vi "HFRR ADV v07.vi"() -> ()   [LabVIEW 2025] (continued)
]]
  out "Residual Uno":string
  out "Residual Due":string
  out "String":string="C:\\Winducom 2010\\1582\\1582\\"
  out "file path":path=path "C:/Windows/wndcm_pw_stdED hfrr.txt"
  out "string":string="49\r50\r51\r10"
  out "x = y?":bool
  out "dipl pwd":string="@143$\n"
  out "string1 4":string
  out "string1 3":string
  out "string1 2":string
  out "string1":string
  out "stopT":bool
  out "Elapsed time 3":dbl=0.10620016403198242 min=0.0 max=6000.0 step=0.01 format="%<%H:%M:%S>t"
  in  "error in (no error)":errorcluster
  out "error out":errorcluster
  in  "RSTCOF 2":bool
  out "PID output":dbl=42.16277107130474 format="%.2f"
  out "Flag":dbl format="%.2f"
  in  "Tab Control 3":enum32{"RMS", "LIVE"}(tab)
  out "array w/ subset deleted":dbl[](array[numeric])
  out "REMARKS":string="@WINDUCOM : RECIPROCATORY TEST RIG    DEFINITON FILE       \r  Sample ID :- , Load :-  2.00 N , Remarks :- , Date :- 05/11/2016, 06:04\r"
  out "Time 2":dbl=0.0004
  in  "reinit":bool=TRUE
  in  "Remarks : 2":string
  out "PID-out":dbl
  out "Rate":dbl=2500.0 caption="Rate (Hz)" min=100.0 max=10000.0 step=1.0
  out "COUNT":i32
  out "FRICVALZ":dbl
  out "Sensor mean 3":dbl
  out "Sensor mean":dbl(slide) min=0.0 max=5.0 step=0.001 scale=0.0..5.0
  out "Sensor mean 2":dbl
  in  "ao0":errorcluster
  out "String 2":string
  out "clk":dbl min=0.0 max=999999999.0 step=0.25 format="%.2f"
  out "spm":string
  out "stp":dbl=0.25 min=0.25 max=60.0 step=0.25 format="%.2f"
  # "© Copyright 2023 | Paltro Inc"
  # "HFRR ADV"
  # "ADV"
  # "Camera Initialization in Progress"
  # "Test Setup"
  # "SAMPLE INFO"
  # "Hz"
  # "grams"
  # "mm"
  # "°C"
  # "%RH"
  # "min"
  # "mins remaining"
  # "°C"
  # "Coefficient of Friction"
  # "Frictional Force ( N )"
  # "Electrical Contact Resistance ( % )"
  # "Temperature ( °C )"
  # "Heater"
  # "( mm )"
  # "Hz"
  # "%Rh"
  # "Stroke ( mm )"
  # "Controller"
  # "%"
  # "N"
  # "deg C"
  # "N"
  # "Automated Scar Detection in Progress"
  # "Zoom Factor"
  # "%"
  # "Tools"
  # "Wear Scar Measurements"
  # "Wear Scar"
  # "Wear Scar"
  # "Wear Scar"
  # "µm"
  # "µm"
  # "µm"
  # "Calibration Centre"
  # "Select a calibration procedure to begin. Each procedure guides you through all required steps."
  # "System Control Commands\nS;1 - Starts the full automation cycle (Runs Priming-humidify till 70RH sequence first, then switches to Maintenance).\nS;0 - Stops the system immediately and enters Standby mode (Safe State: All actuators OFF).\nM;1 - Skips the priming sequence and jumps directly to Maintenance mode (PID control).\nR;1 - Resets the logic state machine and clears all errors, returning to Standby.\nService Mode (Manual Control)\nX;1 - Enters Manual Service Mode. This disables all automatic logic, sensor safety checks, and timers.\nX;0 - Exits Manual Service Mode and returns to Standby (Safe State).\nActuator Commands (Only work after sending X;1)\nP;[0-255] - Sets the Pump PWM. Note that this is Active Low (0 = Max Flow, 255 = Pump OFF).\nF;I;[0-255] - Sets the Intake Fan speed (0 = OFF, 255 = Max Speed).\nF;O;[0-255] - Sets the Exhaust Fan speed (0 = OFF, 255 = Max Speed).\nD;1 - Turns the Dehumidifier Relay ON.\nD;0 - Turns the Dehumidifier Relay OFF."
  # "%RH"
  # "ISO : WS1.4"
  # "Start test and end test log--- done\nDisable heater ON and Humidity ON during the test --- done\ntemprature and ---done\nhumidity reach log\nauto start run true logic and log\nmanual start log once"
  # "Reference Fluid Information"
  # "Note:\nMake sure to place all images in the folder \"C:\\WinDucom\\im\" before clicking on \"Import Image.\""
  # "NOTE:\nPlace all the images in the path \"C:\\WinDucom\\im\" before clicking on Import Image"
  # "Wear Scar Measurements"
  # "Reference Fluid Information"
  # "Graph :"
types:
  T1 = enum32{"Home", "Dashboard", "Imaging", "Report", "Analysis", "About", "Test Setup", "Advance", "Calibration"}
  T2 = enum32{"HOME", "Test Setup", "Acquire", "Adv Scar", "Adv Scar Report", "Compare Files", "Calibration", "About", "Advance", "Mooha"}
  T3 = enum16{"ASTM D6079", "ISO 12156", "CEC F-096-A-06", "Custom"}
  T4 = enum32{"Dashboard 1", "Dashboard 2", "Dashboard 3"}
  T5 = enum32{"COF", "Friction", "ECR", "Temperature", "Humidity", "Stroke"}
  T6 = enum32{"Coefficient Of Friction", "Air Temperature", "Humidity", "Stroke", "Sample Temperature", "Electrical Contact Resistance", "Frequency", "Air Temp vs Rh"}
  T7 = enum32{"Main Tab", "Stroke Calibration", "Friction Force ", "Temperature Calibration"}
  T8 = enum32{"Stroke Calibration", "Friction Calibration", "Temperature Calibration"}
  T9 = enum32{"Gains", "Configuration Parameters", "Temperature Calibration"}
  T10 = enum32{"Stroke Data", "Temperature Calibration", "Friction Force Raw Data"}
  T11 = enum32{"Temp Variables", "Camera", "WO 2465 (1)", "WO 2465 (2)", "WO 2465 (3)"}
  T12 = typedef "Auto Start enum.ctl" = enum16{"Init", "Humidity & Temperature On", "Reach point", "Maintain Stage", "Start Stage", "close", "Exit"}
  T13 = typedef "imagedata.ctl" = cluster{"image type":i32, "image depth":i32, "image":u8[], "mask":u8[], "colors":u32[], "Rectangle":cluster{"left":i16, "top":i16, "right":i16, "bottom":i16}}
  T14 = enum32{"HOME", "Test Setup", "Acquire", "Compare Files", "Print Report", "About", "Advance", "Mooha"}
  T15 = enum8{"Enabled", "Disabled", "Disabled and Grayed Out"}
  T16 = cluster{"Read Heave and Surge":string, "Bytes at Heave Port":dbl, "Heave and Surge COM Port:":refnum<visa-resource-name>, "Com Port 2":refnum<visa-resource-name>, "Residual Due":string, "Heave COM Status 2":bool, "Heave COM Status":bool, "Port 2":bool, "Sway PPR":dbl, "Surge PPR":dbl, "Heave PPR":dbl, "Sway Pitch":dbl, "Surge Pitch":dbl, "Heave Pitch":dbl, "Sway Pulses/mm":dbl, "Surge Pulses/mm":dbl, "Heave Pulses/mm":dbl, "inner loop":dbl, "Read Heave and Surge 2":string, "String 36":string, "Write S":bool, "WriteCC1":string[], "Heave COM Loop":i32, "LastCom":string, "EXIT":bool, "Error Heave":errorcluster}
  T17 = enum32{"HOME", "Test Setup", "Acquire", "Adv Scar", "Adv Scar Report", "Compare Files", "About", "Advance", "Mooha"}
  T18 = enum16{"Always On", "Always Off", "Off While Running"}
  T19 = typedef "POST ANALYSIS ENUM.ctl" = enum16{"OPEN EXE", "INIT", "OPEN FILE", "FIT", "DRAW REC", "DRAW LINE", "PAN", "ZOOM IN", "ZOOM OUT", "SET ZOOM", "CLEAR ROI", "GET MEASUREMENTS", "RESIZE MODE", "STREAM START", "STREAM STOP", "SHOW UI", "MINIMIZE UI", "HIDE UI", "CKISE APP", "CLOSE CONNECTION", "SAVE IMAGE", "SET ROI COLOR", "READ", "TCP CHECK", "CLOSE"}
  T20 = typedef "CAMERA LIVE FEED ENUM.ctl" = enum16{"OPEN EXE", "INIT", "READ", "CAMERA CONNECT", "CAMERA START", "CAMERA STOP", "CAMERA GRAY", "CAMERA RGB", "CAMERA MINIMIZE", "CAMERA CLOSE", "CAMERA MODE LIST", "CAMERA MODE SET", "CAMERA RESTORE", "CAMERA SAVE", "CLOSE"}
  T21 = cluster{"File Name":string, "Test Method":string, "Operator":string, "Fuel Description":string, "Date and time":string}
  T22 = enum32{"Home", "Dashboard", "Imaging", "Report", "Analysis", "About", "Test Setup"}
  T23 = enum32{"HOME", "Test Setup", "Acquire", "Compare Files", "About", "Advance", "Mooha"}
  T24 = enum16{"deny read/write", "deny write-only", "deny none"}
  T25 = typedef "NI_ReportGenerationCore.lvlib/HTML Report Image Alignment.ctl" = enum16{"(default)", "LEFT", "RIGHT", "TOP", "TEXTTOP", "MIDDLE", "ABSMIDDLE", "BASELINE", "BOTTOM", "ABSBOTTOM"}
  T26 = enum32{"Home", "Dashboard", "Imaging", "Report", "Analysis", "About", "Test Setup", "Advance"}
  T27 = enum16{"open", "replace", "create", "open or create", "replace or create", "replace or create with confirmation"}
  T28 = enum16{"INIT", "READ", "MANUAL WRITE", "WRITE", "CLOSE", "ERROR INIT"}
  T29 = enum16{"open", "open or create", "create or replace", "create", "open (read only)"}
  T30 = cluster{"Mode":enum16{"RTU", "ASCII"}, "Slave Address":u8}
diagram:
  w10 = FALSE ("Visible")
  w11 = T15."Enabled" ("Disabled")
  w14 = FALSE ("Visible")
  w13 = FALSE ("Humidity Off Command")
  w31 = "" ("USER ID")
  (unwired) T17."HOME" ("Main Tab")
  # "[CH1]    - FF\n[CH2]   - TEMPERATURE\n[CH3]    - Humidity\n[CH4]    - AIR TEMP\n[CH5]\\- Visa Uno\n[CH6] \\- Visa Due\n[CH7]  \\- file path\n[CH8]   - Displacement Gain\n[CHA]   - Stroke Gain\n[CHB]   - Stroke PID Gain\n[CHC]   -Language Selection\n[CHD]   -Power +\n[CHE]   -Power_\n[CHF]   -Heater\n[CHG]   -Humidity Wet\n[CHH]   -Humidity Dry\n[CHI]   -Integral Time \n[CHIJ   -Air intercept\n[CHI]   -Temp Intercept"
  n1 = flat-sequence {
    tunnel: [w80] -> w23
    tunnel: w23 -> [w94]
    tunnel: [w93] -> w22
    tunnel: ["ao0"] -> w25
    tunnel: w22 -> [_]
    tunnel: w25 -> [w158]
    tunnel: [w158] -> w24
    tunnel: w24 -> [w204]
    tunnel: [w202] -> w35
    tunnel: [w204] -> w34
    tunnel: w35 -> [w254]
    tunnel: w34 -> [w211]
    tunnel: [w254] -> w21
    tunnel: [w217] -> w20
    tunnel: [w205] -> w19
    tunnel: [w260] -> _
    tunnel: [w259] -> _
    tunnel: [w261] -> w57
    tunnel: w21 -> [w261]
    tunnel: w20 -> [w259]
    tunnel: w19 -> [w260]
    frame #0 {
      n2 = disable-structure shown="Disabled" {
        frame Disabled {
          n3 = control-ref of="This VI"() -> (w68:refnum<vi>)
          n4 = property class="VI"(reference=w68) -> (reference out=w59:refnum<vi>, error out=w63:errorcluster, "Panel"=w67:refnum<vi>)  [unwired: 1 in]
          n5 = property class="Pnl"(reference=w67, error in=w63) -> (reference out=w61:refnum<vi>, error out=w64:errorcluster, "Panes[]"=w66:refnum<vi>[])
          n6 = for {
            tunnel: w66 -> [w74] mode=indexing
            tunnel: T18."Always Off" ("Horizontal Scrollbar Visibility") -> [w73]
            tunnel: w64 -> [w70]
            tunnel: [w69] -> w62
            n7 = property class="Pane"(reference=w74, error in=w70, "HorizScrollbarVisibility"=w73) -> (reference out=w71:refnum<vi>, error out=w72:errorcluster)
            n8 = Close Reference(reference=w71, error in (no error)=w72) -> (error out=w69:errorcluster)
          }
          n9 = Close Reference(reference=w61, error in (no error)=w62) -> (error out=w60:errorcluster)
          n10 = Close Reference(reference=w59, error in (no error)=w60) -> (error out=→"error out 8":errorcluster)
        }
        frame Enabled {
        }
      }
    }
    frame #1 {
      n11 = call "CLOSE CONNECTION.vi"("error in (no error)"="error in (no error) 2") -> ("error out"=w78:errorcluster)  [unwired: 10 in]
      n12 = call <vilib>:"Clear Errors.vi"("error in (no error)"=w78) -> ("error out"=w77:errorcluster)  [unwired: 5 in, 1 out]
      n13 = disable-structure shown="Enabled" {
        disable-tunnel: w77 -> [w84 _]
        disable-tunnel: [w83 _] -> w80
        frame Enabled {
          n14 = call <userlib>:"Fit VI window to Largest Dec.vi"("error in (no error)"=w84, "border spacing (2 px)"=1) -> ("error out"=w87:errorcluster, "dup VI Ref"=w91:refnum<vi>)  [unwired: 4 in]
          n15 = invoke on="Invoke Node" class="VI" method="FP.Run-Time Position.Maximized"(reference=w91, error in=w87) -> (error out=w88:errorcluster)  [unwired: 2 in, 3 out]
          n16 = call <vilib>:"Clear Errors.vi"("error in (no error)"=w88) -> ("error out"=w90:errorcluster)  [unwired: 5 in, 1 out]
          n17 = control-ref of="This VI"() -> (w82:refnum<vi>)
          n18 = invoke on="Invoke Node" class="VI" method="Default Vals.Reinit All"(reference=w82, error in=w90) -> (reference out=w86:refnum<vi>, error out=w85:errorcluster)  [unwired: 1 in, 1 out]
          n19 = Close Reference(reference=w86, error in (no error)=w85) -> (error out=w83:errorcluster)
        }
        frame Disabled {
        }
      }
      n20 = local write "sign in temp"(FALSE ("sign in temp")) -> ()
      n21 = property on="Sign In" class="Bool (strict)"("DisabledEnum"=T15."Disabled" ("Disabled")) -> ()  [unwired: 2 in, 2 out]
      n22 = property on="Auto Scar Check" class="Clust (strict)"("Visible"=TRUE) -> ()  [unwired: 2 in, 2 out]
    }
    frame #2 {
      n23 = call "dialog box.vi"("Status"="Before starting the test, verify that the microscope cable is connected.", "error in"=w94) -> ("error out"=w93:errorcluster)  [unwired: 8 in]
    }
    frame #3 {
      (unwired) T17."HOME" ("Main Tab")
      (unwired) TRUE ("Re-Initialise")
      w100 = FALSE ("Upld AR 2")
      # "kkkkk"
      # "C:\\Windows\\wndcm_pw_stdED hfrr.txt"
      # "C:\\LAB-IQ NXT"
      # "C:\\LAB-IQ NXT\\wndcm_pw_stdED hfrr.txt"
      # "password file"
      n24 = Current VI's Path() -> (path=w113:path)
      n25 = Strip Path(path=w113) -> (stripped path=w106:path)  [unwired: 1 out]
      n26 = Path To String(path=w106) -> (string=w108:string)
      n27 = local write "conststatus"(0.0 ("rpm value : 2")) -> ()
      n28 = local write "Upld AR 2"(TRUE ("Upld AR 2")) -> ()
      n29 = local write "FLAG 2"(0.0 ("FLAG 2")) -> ()
      n30 = local write "Com flag"(u32 0 ("Com flag")) -> ()
      n31 = local write "Lan flag"(0.0 ("Lan flag")) -> ()
      n32 = local write "COUNT"(0 ("COUNT")) -> ()
      n33 = local write "refresh flag"(FALSE ("refresh flag")) -> ()
      n34 = local write "Json St Flg"(w100) -> ()
      n35 = Search/Split String(string=w108, search string/char (-)=".exe") -> (match + rest of string=w110:string)  [unwired: 1 in, 2 out]
      n36 = Match True/False String(2:".vi" ("false string"), 3:".exe" ("true string"), 4:w110) -> (0:w107:bool)  [unwired: 1 out]
      n37 = local write "Json End Flg"(w100) -> ()
      n38 = case shown="True" w107 {
        tunnel: w106 -> [w129 w131]
        tunnel: [w129 w130] -> w104
        frame False {
        }
        frame True {
          n39 = Strip Path(path=w131) -> (stripped path=w130:path)  [unwired: 1 out]
        }
      }
      n40 = Path To String(path=w104) -> (string=→"Gain path":string)
      n41 = local write "Main Tab Display"(T4."Dashboard 1" ("Main Tab Display")) -> ()
      n42 = local write "main tab sub"(enum32{"Page 1", "Page 2"}."Page 1" ("main tab sub")) -> ()
      n43 = local write "Main Tab"(T2."HOME" ("Main Tab")) -> ()
      n44 = local write "EVENT LOG"("") -> ()
      n45 = List Folder(path=path "C:/LAB-IQ" ("directory path"), pattern="*.txt") -> (filenames=w119:string[])  [unwired: 2 in, 3 out]
      n46 = Search 1D Array(1D array=w119, element="wndcm_pw_stdED hfrr.txt") -> (index of element=w122:i32)  [unwired: 1 in]
      n47 = Equal?(x=w122, y=-1) -> (x = y?=w117:bool)
      n48 = case shown="True" w117 {
        frame False {
        }
        frame True {
          n49 = String To Byte Array(string="123\n") -> (unsigned byte array=w136:u8[])
          n50 = Array Size(array=w136) -> (size(s)=w135:i32)
          n51 = for {
            N: w135 -> [_]
            tunnel: w136 -> [w149]
            tunnel: [w146] -> w138 mode=indexing
            tunnel: w135 -> [w141]
            i -> [w139]
            n52 = Decrement(x=w141) -> (x-1=w142:i32)
            n53 = Equal?(x=w139, y=w142) -> (x = y?=w143:bool)
            n54 = Index Array(array=w149, index=w139) -> (element=w148:u8)
            n55 = Number To Decimal String(number=w148) -> (decimal integer string=w147:string)  [unwired: 1 in]
            n56 = Select(t="", s=w143, f="\r") -> (s? t:f=w140:string)
            n57 = Concatenate Strings(w147, w140) -> (w146:string)
          }
          n58 = local read "file path"() -> (w132:path)
          n59 = Concatenate Strings(w138) -> (w134:string)
          n60 = call <vilib>:"Write Characters To File.vi"("append to file? (new file:F)"=FALSE, "character string"=w134, "file path (dialog if empty)"=w132) -> ()  [unwired: 2 in, 1 out]
        }
      }
      n61 = local write "clk"(0.0 ("clk")) -> ()
      n62 = local write "Flag"(0.0 ("Flag")) -> ()
      "file path" <- path "C:/LAB-IQ/wndcm_pw_stdED hfrr.txt" ("file path")
      "FF buffer" <- dbl[] [] ("FF buffer")
    }
    frame #4 {
      # "C:\\WinDucom\\calibrate WO 2391.dcf"
      n63 = String To Path(string="C:\\LAB-IQ\\calibrate WO 2465.dcf") -> (path=w157:path)
      n64 = Open/Create/Replace File "Open File"(file path (use dialog)=w157) -> (refnum out=w156:refnum<file>)  [unwired: 5 in, 2 out]
      n65 = for {
        N: 24 -> [_]
        tunnel: w156 -> [w177]
        i -> [w171]
        (unwired) TRUE ("line mode (F)")
        n66 = Read from Text File "Read File"(file (use dialog)=w177) -> (text=w176:string)  [unwired: 3 in, 3 out]
        n67 = Match Pattern(string=w176, regular expression="]") -> (after substring=w174:string)  [unwired: 1 in, 3 out]
        n68 = String Subset(string=w176, offset (0)=5, length (rest)=10 ("length (rest)")) -> (substring=w169:string)
        n69 = Fract/Exp String To Number(string=w169) -> (number=w170:dbl)  [unwired: 3 in, 1 out]
        n70 = Match Pattern(string=w174, regular expression="-") -> (before substring=w172:string)  [unwired: 1 in, 3 out]
        n71 = case shown="20" w171 {
          tunnel: w170 -> [w180 w181 w182 w183 _ _ _ w188 w189 _ w190 w191 w192 w193 w194 w195 _ w196 w197 _ _ _ _ _ _]
          tunnel: w172 -> [_ _ _ _ w184 w185 w186 _ _ _ _ _ _ _ _ _ _ _ _ w198 w199 _ w200 w201 _]
          frame 0 {
            n72 = local write "FRIC. FORCE :"(w180) -> ()
          }
          frame 1 {
            n73 = local write "TEMPERATURE :"(w181) -> ()
          }
          frame 2 {
            n74 = local write "HUMIDITY:"(w182) -> ()
          }
          frame 3 {
            n75 = local write "AIR TEMPERATURE :"(w183) -> ()
          }
          frame 4 {
            n76 = local write "Com Port 1"(w184) -> ()
          }
          frame 5 {
            n77 = local write "Com Port 2"(w185) -> ()
            n78 = local write "visa due"(w185) -> ()
          }
          frame 6 {
            n79 = String To Path(string=w186) -> (path=w187:path)
            n80 = local write "File Path"(w187) -> ()
          }
          frame 7 {
            n81 = local write "DISPLACEMENT :"(w188) -> ()
          }
          frame 8 {
            n82 = local write "STROKE GAIN :"(w189) -> ()
          }
          frame 9 {
          }
          frame 10 {
            n83 = local write "Language Selection"(w190) -> ()
          }
          frame 11 {
            n84 = local write "CH-POWER +"(w191) -> ()
          }
          frame 12 {
            n85 = local write "CH-POWER -"(w192) -> ()
          }
          frame 13 {
            n86 = local write "CH-HEATER"(w193) -> ()
          }
          frame 14 {
            n87 = local write "CH-HUMIDITY WET"(w194) -> ()
          }
          frame 15 {
            n88 = local write "CH-HUMIDITY DRY"(w195) -> ()
          }
          frame 16 {
          }
          frame 17 {
            n89 = local write "AIR TEMP INTERCEPT:"(w196) -> ()
          }
          frame 18 {
            n90 = local write "TEMP INTERCEPT:"(w197) -> ()
          }
          frame 19 {
            n91 = local write "S.NO"(w198) -> ()
          }
          frame 20 {
            n92 = local write "Com Port 3"(w199) -> ()
          }
          frame 21 {
          }
          frame 22 {
            n93 = local write "C3 :"(w200) -> ()
          }
          frame 23 {
            n94 = local write "Camera Port :"(w201) -> ()
          }
          frame 24, Default {
          }
        }
      }
      n95 = String To Path(string="C:\\LAB-IQ\\Image Calibrate v01.dcf") -> (path=w153:path)
      n96 = Open/Create/Replace File ("Open File")(file path (use dialog)=w153) -> (refnum out=w152:refnum<file>)  [unwired: 5 in, 2 out]
      n97 = for {
        N: 4 -> [_]
        tunnel: w152 -> [w164]
        i -> [w160]
        n98 = Read from Text File ("Read File")(file (use dialog)=w164) -> (text=w165:string)  [unwired: 3 in, 3 out]
        n99 = String Subset(string=w165, offset (0)=6, length (rest)=10 ("length (rest)")) -> (substring=w161:string)
        n100 = Fract/Exp String To Number(string=w161) -> (number=w159:dbl)  [unwired: 3 in, 1 out]
        n101 = case shown="3" w160 {
          tunnel: w159 -> [w166 w167 _ w168 _]
          frame 0 {
            n102 = local write "5x Gain"(w166) -> ()
          }
          frame 1 {
            n103 = local write "10x Gain"(w167) -> ()
          }
          frame 2 {
          }
          frame 3 {
            n104 = local write "100x gain"(w168) -> ()
          }
          frame 4, Default {
          }
        }
      }
    }
    frame #5 {
      n105 = Wait (ms)(milliseconds to wait=u32 1000) -> (millisecond timer value=w202:u32)
    }
    frame #6 {
      w220 = u32 2000 ("milliseconds to wait")
      w247 = u32 2000 ("milliseconds to wait")
      n106 = call "CAMERA LIVE FEED FGV.vi"("Enum - Menu"=CAMERA_LIVE_FEED_ENUM."OPEN EXE", "error in (no error)"=w211) -> ("error out"=w253:errorcluster)  [unwired: 8 in, 1 out]
      n107 = call "Stall Data Flow.vim"("value in"=w253, "milliseconds to wait"=w247) -> ("value out"=w251:errorcluster)  [unwired: 1 out]
      n108 = call "CAMERA LIVE FEED FGV.vi"("Enum - Menu"=CAMERA_LIVE_FEED_ENUM."INIT", "error in (no error)"=w251) -> ("error out"=w249:errorcluster)  [unwired: 8 in, 1 out]
      n109 = call "IMAGE ANALYSIS.vi"("Enum"=POST_ANALYSIS_ENUM."OPEN EXE", "error in"=w211) -> ("error out"=w208:errorcluster)  [unwired: 8 in, 1 out]
      n110 = call "Stall Data Flow.vim"("value in"=w208, "milliseconds to wait"=u32 8000) -> ("value out"=w207:errorcluster)  [unwired: 1 out]
      n111 = property on="Camera Port :" class="CmbBox"() -> ("Strings[]"=w245:string[], "Value"=w246:string)  [unwired: 2 in, 2 out]
      n112 = call "IMAGE ANALYSIS.vi"("Enum"=POST_ANALYSIS_ENUM."INIT", "error in"=w207) -> ("error out"=w205:errorcluster)  [unwired: 8 in, 1 out]
      n113 = Search 1D Array(1D array=w245, element=w246) -> (index of element=w244:i32)  [unwired: 1 in]
      n114 = case shown="Error .." w249 {
        selector: w249 -> [w255 _]
        tunnel: [w255 _] -> w248
        frame No Error {
        }
        frame Error {
          n115 = One Button Dialog(message="Camera initialization error.\nPlease Restart the software") -> ()  [unwired: 1 in, 1 out]
        }
      }
      n116 = Type Cast(type=30, x=w244) -> (*(type *) &x=w242:i32)
      n117 = call "Stall Data Flow.vim"("value in"=w248, "milliseconds to wait"=w247) -> ("value out"=w224:errorcluster)  [unwired: 1 out]
      n118 = Add(x=w242, y=48) -> (x+y=w223:i32)
      n119 = call "CAMERA LIVE FEED FGV.vi"("Enum - Menu"=CAMERA_LIVE_FEED_ENUM."CAMERA CONNECT", "error in (no error)"=w224, "CAMERA PORT"=w223) -> ("error out"=w233:errorcluster)  [unwired: 7 in, 1 out]
      n120 = call "Stall Data Flow.vim"("value in"=w233, "milliseconds to wait"=u32 5000) -> ("value out"=w234:errorcluster)  [unwired: 1 out]
      n121 = call "CAMERA LIVE FEED FGV.vi"("Enum - Menu"=CAMERA_LIVE_FEED_ENUM."CAMERA MODE LIST", "error in (no error)"=w234) -> ("error out"=w236:errorcluster)  [unwired: 8 in, 1 out]
      n122 = call "Stall Data Flow.vim"("value in"=w236, "milliseconds to wait"=w220) -> ("value out"=w235:errorcluster)  [unwired: 1 out]
      n123 = call "CAMERA LIVE FEED FGV.vi"("Enum - Menu"=CAMERA_LIVE_FEED_ENUM."READ", "error in (no error)"=w235) -> ("error out"=w222:errorcluster, "data out"=→"Camera List":string)  [unwired: 8 in]
      n124 = Type Cast(type=30, x=0) -> (*(type *) &x=w216:i32)
      n125 = call "Stall Data Flow.vim"("value in"=w222, "milliseconds to wait"=w220) -> ("value out"=w221:errorcluster)  [unwired: 1 out]
      n126 = Add(x=w216, y=48) -> (x+y=w214:i32)
      n127 = call "CAMERA LIVE FEED FGV.vi"("Enum - Menu"=CAMERA_LIVE_FEED_ENUM."CAMERA MODE SET", "error in (no error)"=w221, "CAMERA MODE"=w214) -> ("error out"=w218:errorcluster)  [unwired: 7 in, 1 out]
      n128 = call "Stall Data Flow.vim"("value in"=w218, "milliseconds to wait"=u32 2000) -> ("value out"=w238:errorcluster)  [unwired: 1 out]
      n129 = call "CAMERA LIVE FEED FGV.vi"("Enum - Menu"=CAMERA_LIVE_FEED_ENUM."CAMERA START", "error in (no error)"=w238) -> ("error out"=w239:errorcluster)  [unwired: 8 in, 1 out]
      n130 = call "Stall Data Flow.vim"("value in"=w239, "milliseconds to wait"=u32 1000) -> ("value out"=w240:errorcluster)  [unwired: 1 out]
      n131 = call "CAMERA LIVE FEED FGV.vi"("Enum - Menu"=CAMERA_LIVE_FEED_ENUM."CAMERA MINIMIZE", "error in (no error)"=w240) -> ("error out"=w217:errorcluster)  [unwired: 8 in, 1 out]
    }
    frame #7 {
      n132 = case shown="No Error" w259 {
        frame No Error {
          n133 = property on="Auto Scar Check" class="Clust (strict)"("Visible"=FALSE) -> ()  [unwired: 2 in, 2 out]
        }
        frame Error {
        }
      }
      n134 = local write "sign in temp"(TRUE ("sign in temp")) -> ()
      n135 = property on="Sign In" class="Bool (strict)"("DisabledEnum"=T15."Enabled" ("Disabled")) -> ()  [unwired: 2 in, 2 out]
    }
  }
  n136 = local write "Cal Password"("" ("Cal Password")) -> ()
  n137 = property on="Auto Start Test" class="Bool (strict)"("Visible"=TRUE) -> ()  [unwired: 2 in, 2 out]
  n138 = property on="FRICVALZ 4" class="Bool (strict)"("DisabledEnum"=w11) -> ()  [unwired: 2 in, 2 out]
  n139 = property on="FRICVALZ 2" class="Bool (strict)"("DisabledEnum"=w11) -> ()  [unwired: 2 in, 2 out]
  n140 = property on="FRICVALZ 3" class="Bool (strict)"("DisabledEnum"=w11) -> ()  [unwired: 2 in, 2 out]
  n141 = property on="About" class="Clust (strict)"("Visible"=FALSE) -> ()  [unwired: 2 in, 2 out]
  n142 = property on="Tab Control 5" class="TabCtl (strict)"("Tabs Visible?"=TRUE ("Page Labels Display Visible?")) -> ()  [unwired: 2 in, 2 out]
  n143 = property on="Wrong Password" class="Str"("Visible"=w10) -> ()  [unwired: 2 in, 2 out]
  n144 = property on="Calibration 2" class="TabCtl (strict)"("Visible"=w10) -> ()  [unwired: 2 in, 2 out]
  n145 = local write "SCAR MEASURMENT"(enum32{"Auto Scar", "Manual Scar"}."Manual Scar" ("SCAR MEASURMENT")) -> ()
  n146 = local write "Temperature Off Command"(w13) -> ()
  n147 = local write "Main Dashboard Buttons"(T1."Home" ("Main Dashboard Buttons")) -> ()
  n148 = local write "Humidity Off Command"(w13) -> ()
  n149 = local write "CAMERA ROI MIN TEMP"(w13) -> ()
  n150 = local write "TEST FILE NAM,E SAVED"(w13) -> ()
  n151 = local write "LIVE FEED MIN TEMP"(w13) -> ()
  n152 = local write "SCAR MEASURMENT"(enum32{"Auto Scar", "Manual Scar"}."Manual Scar" ("SCAR MEASURMENT")) -> ()
  n153 = while {
    stop <- w263 stop-if-true
    n154 = event shown="[1] \"RUN\": Value Change" {
      selector: _ -> [_ _ _ _ _ _ _ _ _ _ _ _ _ _]
      dyn-events: _ -> [_ _ _ _ _ _ _ _ _ _ _ _ _ _]
      timeout: 100 -> [_ _ _ _ _ _ _ _ _ _ _ _ _ _]
      tunnel: [FALSE FALSE _ FALSE _ _ _ _ _ _ _ _ _ TRUE] -> w263
      event Timeout {
        n155 = event-data() -> ()  [unwired: 1 in, 3 out]
        n156 = disable-structure shown="Disabled" {
          frame Disabled {
            n157 = local read "Auto Start Test"() -> (w277:bool)
            n158 = local read "RUN"() -> (w278:bool)
            n159 = Or(x=w278, y=w277) -> (x .or. y?=w276:bool)
            n160 = case shown="True" w276 {
              frame False {
                w279 = TRUE ("PAUSE")
                n161 = call "ELAPSED TIMER VI - abort test.vi"("RESET"=w279, "PAUSE"=w279) -> ()  [unwired: 7 in, 3 out]
              }
              frame True {
                n162 = local read "Stroke 2"() -> (w284:dbl)
                n163 = local read "FF 3"() -> (w286:dbl)
                n164 = Equal?(x=w284, y=0.95 ("Stroke 2")) -> (x = y?=w281:bool)
                n165 = Equal?(x=w286, y=0.0 ("FF 3")) -> (x = y?=w282:bool)
                n166 = Or(x=w282, y=w281) -> (x .or. y?=w280:bool)
                n167 = case shown="True" w280 {
                  selector: w280 -> [_ w291]
                  frame False {
                    w287 = TRUE ("PAUSE")
                    n168 = call "ELAPSED TIMER VI - abort test.vi"("RESET"=w287, "PAUSE"=w287) -> ()  [unwired: 7 in, 3 out]
                  }
                  frame True {
                    n169 = Not(x=w291) -> (.not. x?=w290:bool)
                    n170 = call "ELAPSED TIMER VI - abort test.vi"("TARGET"=60.0, "RESET"=w290, "PAUSE"=FALSE) -> ("ELAPSED INDICATION"=w288:bool)  [unwired: 6 in, 2 out]
                    n171 = case shown="True" w288 {
                      frame False {
                      }
                      frame True {
                        n172 = stacked-sequence {
                          frame #0 {
                            w293 = FALSE
                            n173 = local write "Auto Start Test"(w293) -> ()
                            n174 = local write "RUN"(w293) -> ()
                          }
                          frame #1 {
                            n175 = One Button Dialog(message="Test stopped due to a communication error. Reconnect the C1 and C2 cables.") -> ()  [unwired: 1 in, 1 out]
                          }
                        }
                      }
                    }
                  }
                }
              }
            }
          }
          frame Enabled {
          }
        }
        n176 = Get Date/Time In Seconds() -> (seconds since 1Jan1904=w274:timestamp)
        n177 = Format Into String(format string="%<%I:%M:%S:%p %d:%B:%Y>T", w274) -> (resulting string=→"Time Stamp":string)  [unwired: 2 in, 1 out]
        n178 = local read "Service Password enable"() -> (w266:bool)
        n179 = local read "FILE"() -> (w271:string)
        n180 = call <vilib>:"Trim Whitespace.vi"("string"=w271) -> ("trimmed string"=w270:string)  [unwired: 1 in]
        n181 = String Length(string=w270) -> (length=w269:i32)
        n182 = Greater?(x=w269, y=1) -> (0:w267:bool)
        n183 = case shown="False" w267 {
          tunnel: w266 -> [w295 _]
          frame False {
            n184 = case shown="True" w295 {
              frame True {
                w296 = "Test Start In Service Mode" ("Tip Strip")
                w297 = T15."Enabled" ("Disabled")
                n185 = property on="Auto Start Test" class="Bool (strict)"("DisabledEnum"=w297, "TipStrip"=w296) -> ()  [unwired: 2 in, 2 out]
                n186 = property on="RUN" class="Bool (strict)"("DisabledEnum"=w297, "TipStrip"=w296) -> ()  [unwired: 2 in, 2 out]
              }
              frame False {
                w298 = "Enter File Name to Start Test" ("Tip Strip")
                w299 = T15."Disabled and Grayed Out" ("Disabled")
                n187 = property on="Auto Start Test" class="Bool (strict)"("DisabledEnum"=w299, "TipStrip"=w298) -> ()  [unwired: 2 in, 2 out]
                n188 = property on="RUN" class="Bool (strict)"("DisabledEnum"=w299, "TipStrip"=w298) -> ()  [unwired: 2 in, 2 out]
              }
            }
          }
          frame True {
            w300 = "" ("Tip Strip")
            w301 = T15."Enabled" ("Disabled")
            n189 = property on="Auto Start Test" class="Bool (strict)"("DisabledEnum"=w301, "TipStrip"=w300) -> ()  [unwired: 2 in, 2 out]
            n190 = property on="RUN" class="Bool (strict)"("DisabledEnum"=w301, "TipStrip"=w300) -> ()  [unwired: 2 in, 2 out]
          }
        }
      }
      event "RUN": Value Change {
        n191 = event-data() -> ()  [unwired: 1 in, 6 out]
        n192 = local read "RUN"() -> (w303:bool)
        n193 = case shown="False" w303 {
          frame False {
            n194 = flat-sequence {
              frame #0 {
                n195 = local write "START TEMP"(FALSE ("START TEMP")) -> ()
              }
              frame #1 {
                n196 = Wait (ms)(milliseconds to wait=u32 1500) -> ()  [unwired: 1 out]
              }
              frame #2 {
                w309 = T15."Enabled" ("Disabled")
                w311 = "" ("FILE")
                n197 = local write "Command"("VC;0") -> ()
                n198 = local write "FILE"(w311) -> ()
                n199 = local write "Batch Ref Num :"(w311) -> ()
                n200 = local write "Fuel Discription :"(w311) -> ()
                n201 = local write "Main Tab"(T2."Adv Scar" ("Main Tab")) -> ()
                n202 = local write "Remarks :"(w311) -> ()
                n203 = local write "Main Dashboard Buttons"(T1."Imaging" ("Main Dashboard Buttons")) -> ()
                n204 = local write "TEST FILE NAM,E SAVED"(FALSE ("TEST FILE NAM,E SAVED")) -> ()
                n205 = property on="Stroke ( mm )" class="WFChart (strict)"("History Data"=cluster{"y":dbl, dbl, "y":dbl}[] []) -> ()  [unwired: 2 in, 2 out]
                n206 = property on="Auto Start Test" class="Bool (strict)"("Visible"=TRUE) -> ()  [unwired: 2 in, 2 out]
                n207 = property on="FRICVALZ 4" class="Bool (strict)"("DisabledEnum"=w309) -> ()  [unwired: 2 in, 2 out]
                n208 = property on="FRICVALZ 2" class="Bool (strict)"("DisabledEnum"=w309) -> ()  [unwired: 2 in, 2 out]
                n209 = property on="FRICVALZ 3" class="Bool (strict)"("DisabledEnum"=w309) -> ()  [unwired: 2 in, 2 out]
              }
            }
          }
          frame True {
            n210 = flat-sequence {
              frame #0 {
                n211 = local write "Command"("VC;1") -> ()
              }
              frame #1 {
                n212 = Wait (ms)(milliseconds to wait=u32 2000) -> ()  [unwired: 1 out]
              }
              frame #2 {
                w317 = T15."Disabled" ("Disabled")
                n213 = property on="Auto Start Test" class="Bool (strict)"("Visible"=FALSE) -> ()  [unwired: 2 in, 2 out]
                n214 = local write "START TEMP"(TRUE ("START TEMP")) -> ()
                n215 = property on="FRICVALZ 4" class="Bool (strict)"("DisabledEnum"=w317) -> ()  [unwired: 2 in, 2 out]
                n216 = property on="FRICVALZ 2" class="Bool (strict)"("DisabledEnum"=w317) -> ()  [unwired: 2 in, 2 out]
                n217 = property on="FRICVALZ 3" class="Bool (strict)"("DisabledEnum"=w317) -> ()  [unwired: 2 in, 2 out]
              }
            }
          }
        }
      }
      event "Auto": Value Change {
        n218 = event-data() -> ()  [unwired: 1 in, 6 out]
        n219 = stacked-sequence {
          frame #0 {
            n220 = local write "FILE"("") -> ()
          }
          frame #1 {
            n221 = Get Date/Time In Seconds() -> (seconds since 1Jan1904=w323:timestamp)
            n222 = Format Into String(format string="%<%I_%M_%S_%p_%d_%B_%Y>T", w323) -> (resulting string=w322:string)  [unwired: 2 in, 1 out]
            n223 = local write "FILE"(w322) -> ()
          }
        }
        n224 = local read "Auto"() -> (w320:bool)
        n225 = Not(x=w320) -> (.not. x?=w319:bool)
        n226 = local write "Auto"(w319) -> ()
      }
      event "Auto Start Test": Value Change {
        n227 = event-data() -> ()  [unwired: 1 in, 6 out]
        n228 = local read "Auto Start Test"() -> (w326:bool)
        n229 = case shown="False" w326 {
          frame False {
            n230 = flat-sequence {
              frame #0 {
                n231 = local write "START TEMP"(FALSE ("START TEMP")) -> ()
              }
              frame #1 {
                n232 = Wait (ms)(milliseconds to wait=u32 2000) -> ()  [unwired: 1 out]
              }
              frame #2 {
                w333 = T15."Enabled" ("Disabled")
                w334 = "" ("FILE")
                n233 = local write "Main Tab"(T2."Adv Scar" ("Main Tab")) -> ()
                n234 = local write "Main Dashboard Buttons"(T1."Imaging" ("Main Dashboard Buttons")) -> ()
                n235 = property on="RUN" class="Bool (strict)"("Visible"=TRUE) -> ()  [unwired: 2 in, 2 out]
                n236 = local write "Command"("VC;0") -> ()
                n237 = local write "TEST FILE NAM,E SAVED"(FALSE ("TEST FILE NAM,E SAVED")) -> ()
                n238 = local write "Fuel Discription :"(w334) -> ()
                n239 = local write "Batch Ref Num :"(w334) -> ()
                n240 = local write "Remarks :"(w334) -> ()
                n241 = local write "FILE"(w334) -> ()
                n242 = property on="FRICVALZ 4" class="Bool (strict)"("DisabledEnum"=w333) -> ()  [unwired: 2 in, 2 out]
                n243 = property on="FRICVALZ 2" class="Bool (strict)"("DisabledEnum"=w333) -> ()  [unwired: 2 in, 2 out]
                n244 = property on="FRICVALZ 3" class="Bool (strict)"("DisabledEnum"=w333) -> ()  [unwired: 2 in, 2 out]
              }
            }
          }
          frame True {
            n245 = flat-sequence {
              frame #0 {
                n246 = local write "Command"("VC;1") -> ()
              }
              frame #1 {
                n247 = Wait (ms)(milliseconds to wait=u32 2000) -> ()  [unwired: 1 out]
              }
              frame #2 {
                w339 = T15."Disabled" ("Disabled")
                n248 = property on="RUN" class="Bool (strict)"("Visible"=FALSE) -> ()  [unwired: 2 in, 2 out]
                n249 = property on="FRICVALZ 4" class="Bool (strict)"("DisabledEnum"=w339) -> ()  [unwired: 2 in, 2 out]
                n250 = property on="FRICVALZ 2" class="Bool (strict)"("DisabledEnum"=w339) -> ()  [unwired: 2 in, 2 out]
                n251 = property on="FRICVALZ 3" class="Bool (strict)"("DisabledEnum"=w339) -> ()  [unwired: 2 in, 2 out]
                "START TEMP" <- TRUE
              }
            }
          }
        }
      }
      event "Heater Button": Value Change {
        n252 = event-data() -> ()  [unwired: 1 in, 6 out]
        n253 = local read "Heater Button"() -> (w341:bool)
        n254 = case shown="True" w341 {
          frame False {
            n255 = stacked-sequence {
              frame #0 {
                n256 = Number To Fractional String(number=0.0, precision (6)=i16 2) -> (F-format string=w344:string)  [unwired: 2 in]
                n257 = Concatenate Strings("ST;", w344) -> (w346:string)
                n258 = local write "Command"(w346) -> ()
              }
              frame #1 {
                n259 = Wait (ms)(milliseconds to wait=u32 1500) -> ()  [unwired: 1 out]
              }
              frame #2 {
                n260 = local write "Command"("HE;0" ("Command")) -> ()
              }
              frame #3 {
                n261 = Wait (ms)(milliseconds to wait=u32 1500) -> ()  [unwired: 1 out]
              }
            }
          }
          frame True {
            n262 = stacked-sequence {
              frame #0 {
                n263 = local read "Set Temp"() -> (w351:dbl)
                n264 = Number To Fractional String(number=w351, precision (6)=i16 2) -> (F-format string=w352:string)  [unwired: 2 in]
                n265 = Concatenate Strings("ST;", w352) -> (w354:string)
                n266 = local write "Command"(w354) -> ()
              }
              frame #1 {
                n267 = Wait (ms)(milliseconds to wait=u32 1500) -> ()  [unwired: 1 out]
              }
              frame #2 {
                n268 = local write "Command"("HE;1" ("Command")) -> ()
              }
              frame #3 {
                n269 = Wait (ms)(milliseconds to wait=u32 1500) -> ()  [unwired: 1 out]
              }
            }
          }
        }
      }
      event "FILE", "USERNAME", "USER ID": Mouse Enter {
        n270 = event-data() -> ()  [unwired: 1 in, 4 out]
        n271 = dll-call lib="kernel32.dll" fn="Wow64DisableWow64FsRedirection"("OldValue"=0) -> (error out=w363:errorcluster, "OldValue"=w361:i32)  [unwired: 4 in, 1 out]
        n272 = call <vilib>:"System Exec.vi"("run minimized? (F)"=TRUE, "error in (no error)"=w363, "command line"="C:\\Program Files\\Common Files\\Microsoft Shared\\Ink\\TabTip.exe") -> ("error out"=w362:errorcluster)  [unwired: 5 in, 3 out]
        n273 = dll-call lib="kernel32.dll" fn="Wow64EnableWow64FsRedirection"(error in=w362, "OldValue"=w361) -> ()  [unwired: 4 in, 2 out]
      }
      event "EDIT": Value Change {
        n274 = event-data() -> ()  [unwired: 1 in, 6 out]
        n275 = local read "EDIT"() -> (w364:bool)
        n276 = case shown="False" w364 {
          frame False {
            n277 = control-ref of="This VI"() -> (w381:refnum<vi>)
            n278 = property class="VI"(reference=w381) -> (reference out=w372:refnum<vi>, error out=w376:errorcluster, "Panel"=w380:refnum<vi>)  [unwired: 1 in]
            n279 = property class="Pnl"(reference=w380, error in=w376) -> (reference out=w374:refnum<vi>, error out=w377:errorcluster, "Panes[]"=w379:refnum<vi>[])
            n280 = for {
              tunnel: w379 -> [w387] mode=indexing
              tunnel: T18."Always Off" ("Horizontal Scrollbar Visibility") -> [w386]
              tunnel: w377 -> [w383]
              tunnel: [w382] -> w375
              n281 = property class="Pane"(reference=w387, error in=w383, "HorizScrollbarVisibility"=w386) -> (reference out=w384:refnum<vi>, error out=w385:errorcluster)
              n282 = Close Reference(reference=w384, error in (no error)=w385) -> (error out=w382:errorcluster)
            }
            n283 = Close Reference(reference=w374, error in (no error)=w375) -> (error out=w373:errorcluster)
            n284 = Close Reference(reference=w372, error in (no error)=w373) -> (error out=w367:errorcluster)
            "error out 7" <- w367
            n285 = call <vilib>:"Clear Errors.vi"("error in (no error)"=w367) -> ("error out"=w366:errorcluster)  [unwired: 5 in, 1 out]
